vi "Get Calibration.vi"(0 "Level in":refnum<class "Level.lvclass">, 7 "Fs (Hz)":dbl, 11 "error in (no error)":errorcluster) -> (4 "Level out":refnum<class "Level.lvclass">, 6 "Freq (Hz)":dbl[](array[numeric]), 8 "Mag (dB SPL)":dbl[](array[numeric]), 10 "Phase (degrees)":dbl[](array[numeric]), 15 "error out":errorcluster)   [LabVIEW 2015, in "Level.lvclass"]
uses:
  Level.lvclass
  Level.lvclass/Level.ctl
  Read cal.vi
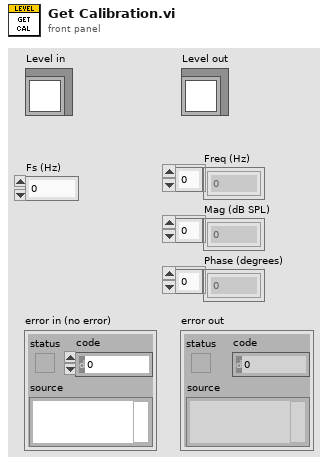
[diagram p1: front panel]
types:
  T1 = cluster{"Freq (Hz)":dbl[], "Mag (dB SPL)":dbl[], "Phase (deg)":dbl[]}
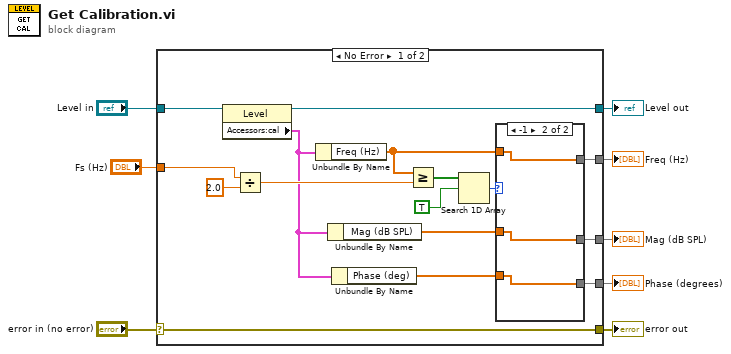
[diagram p0: block diagram]
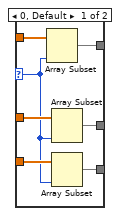
[diagram p2: hidden frame]
diagram:
  n1 = case shown="No Error" "error in (no error)" {
    selector: "error in (no error)" -> [w23 w36]
    tunnel: [w23 w36] -> w7
    tunnel: [w22 w35] -> w5
    tunnel: "Level in" -> [w24 w35]
    tunnel: "Fs (Hz)" -> [w20 _]
    tunnel: [w12 _] -> w3
    tunnel: [w11 _] -> w2
    tunnel: [w10 _] -> w1
    frame No Error {
      n2 = property class="Level"(reference=w24) -> (reference out=w22:refnum<class "Level.lvclass">, "Accessors:cal"=w13:T1)  [unwired: 1 in, 1 out]
      n3 = Divide(x=w20, y=2.0) -> (x/y=w19:dbl)
      n4 = Unbundle By Name(w13) -> ("Freq (Hz)"=w16:dbl[])
      n5 = Unbundle By Name(w13) -> ("Mag (dB SPL)"=w15:dbl[])
      n6 = Unbundle By Name(w13) -> ("Phase (deg)"=w14:dbl[])
      n7 = Greater Or Equal?(x=w16, y=w19) -> (x >= y?=w18:bool[])
      n8 = Search 1D Array(1D array=w18, element=TRUE) -> (index of element=w9:i32)  [unwired: 1 in]
      n9 = case shown="-1" w9 {
        selector: w9 -> [w25 _]
        tunnel: w16 -> [w31 w34]
        tunnel: w15 -> [w30 w33]
        tunnel: w14 -> [w29 w32]
        tunnel: [w28 w34] -> w12
        tunnel: [w27 w33] -> w11
        tunnel: [w26 w32] -> w10
        frame 0, Default {
          n10 = Array Subset(array=w31, length=w25) -> (w28:dbl[])  [unwired: 1 in]
          n11 = Array Subset(array=w30, length=w25) -> (w27:dbl[])  [unwired: 1 in]
          n12 = Array Subset(array=w29, length=w25) -> (w26:dbl[])  [unwired: 1 in]
        }
        frame -1 {
        }
      }
    }
    frame Error {
    }
  }
  "error out" <- w7
  "Level out" <- w5
  "Freq (Hz)" <- w3
  "Mag (dB SPL)" <- w2
  "Phase (degrees)" <- w1
